vi "Read rioConfig.vi"(8 "error in (no error)":errorcluster, 11 "RIOHandler in":refnum<class "RIOHandler.lvclass">) -> (0 "error out":errorcluster, 2 "RIOConfig.lvclass":refnum<class "RIOConfig.lvclass">, 3 "RIOHandler out":refnum<class "RIOHandler.lvclass">)   [LabVIEW 2013, in "ComponentData.lvlib" / "RIOHandler.lvclass"]
uses:
  <userlib>/Common/Component/Application/RT/ComponentData/RIOHandler/RIOHandler.lvclass
  <userlib>/Common/Component/Application/RT/ComponentData/ConfigurationHandler/RIOConfig/RIOConfig.lvclass
  <userlib>/Common/Component/Application/RT/ComponentData/RIOHandler/RIOHandler.lvclass/RIOHandler.ctl
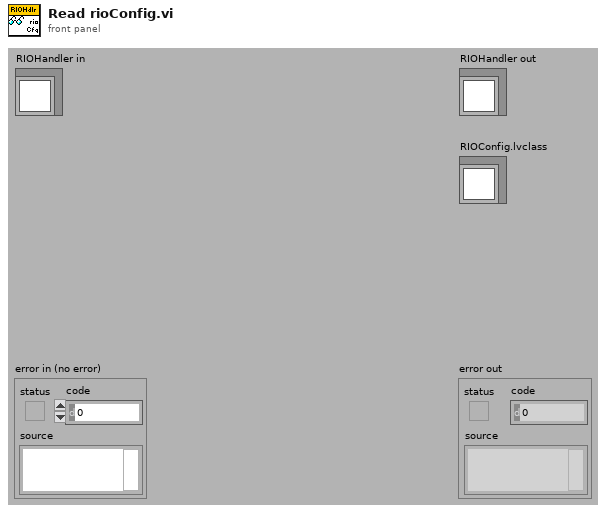
[diagram p1: front panel]
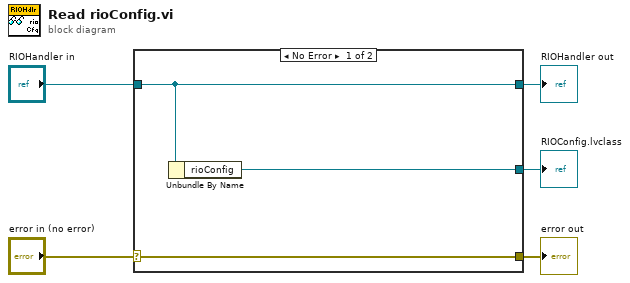
[diagram p0: block diagram]
diagram:
  n1 = case shown="No Error" "error in (no error)" {
    selector: "error in (no error)" -> [w8 w9]
    tunnel: [w8 w9] -> w4
    tunnel: [w7 w10] -> w2
    tunnel: "RIOHandler in" -> [w7 w10]
    tunnel: [w6 _] -> w1
    frame No Error {
      n2 = Unbundle By Name(w7) -> ("rioConfig"=w6:refnum<class "RIOConfig.lvclass">)
    }
    frame Error {
    }
  }
  "error out" <- w4
  "RIOHandler out" <- w2
  "RIOConfig.lvclass" <- w1
